vi "m1m3_issueCommand_ApplyAOSCorrectionByBendingModes.vi"(8 "error in (no error)":errorcluster, 11 "command_ApplyAOSCorrectionByBendingModes_Ctl":T1={"Coefficients[22]"=[0.0, 0.0, 0.0, 0.0, 0.0, 0.0, 0.0, 0.0, 0.0, 0.0, 0.0, 0.0, 0.0, 0.0, 0.0, 0.0, 0.0, 0.0, 0.0, 0.0, 0.0, 0.0]}) -> (0 "error out":errorcluster, 2 "function return":i32, 3 "command_ApplyAOSCorrectionByBendingModes_Ctl out":T1)   [LabVIEW 2016, in "SALLV_m1m3.lvlib"]
doc: "int m1m3_shm_issueCommand_ApplyAOSCorrectionByBendingModesLV(m1m3_command_ApplyAOSCorrectionByBendingModesLV *command_ApplyAOSCorrectionByBendingModes_Ctl );"
uses:
  SALLV_m1m3.lvlib
  DataTypes/command_ApplyAOSCorrectionByBendingModes.ctl
  SALLV_m1m3.so
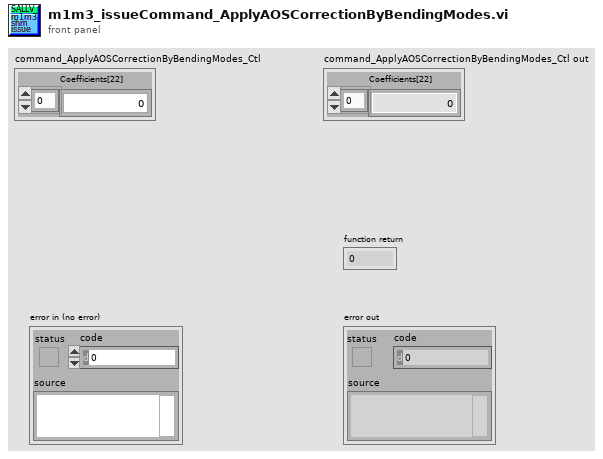
[diagram p1: front panel]
types:
  T1 = typedef "SALLV_m1m3.lvlib/command_ApplyAOSCorrectionByBendingModes.ctl" = cluster{"Coefficients[22]":dbl[]}
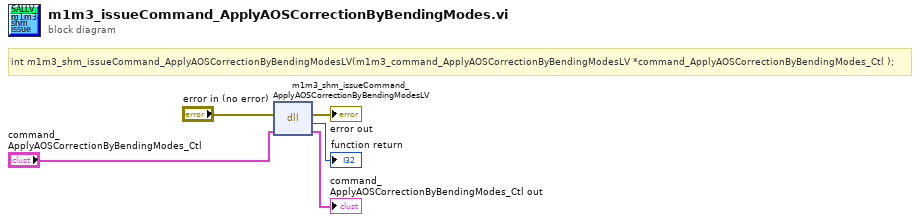
[diagram p0: block diagram]
diagram:
  # "int m1m3_shm_issueCommand_ApplyAOSCorrectionByBendingModesLV(m1m3_command_ApplyAOSCorrectionByBendingModesLV *command_ApplyAOSCorrectionByBendingModes_Ctl );"
  n1 = dll-call lib="opt/CODE/SALLV_m1m3/SALLV_m1m3.*" fn="m1m3_shm_issueCommand_ApplyAOSCorrectionByBendingModesLV"(error in="error in (no error)", "command_ApplyAOSCorrectionByBendingModes_Ctl"="command_ApplyAOSCorrectionByBendingModes_Ctl") -> (error out=→"error out":errorcluster, →"function return":i32, "command_ApplyAOSCorrectionByBendingModes_Ctl"=→"command_ApplyAOSCorrectionByBendingModes_Ctl out":T1)  [unwired: 2 in, 1 out]
